vi "ClearSession.vi"(8 "error in (no error)":errorcluster, 11 "Python in":T2) -> (0 "error out":errorcluster, 3 "Arduino":T1)   [LabVIEW 2021]
uses:
  PythonCtrl.ctl
  Processors.ctl
  ArduinoCtrl.ctl
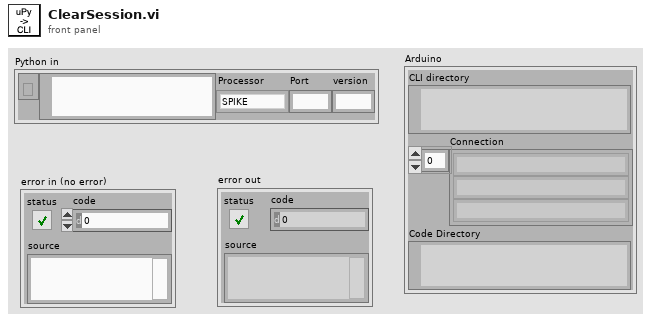
[diagram p1: front panel]
types:
  T1 = typedef "ArduinoCtrl.ctl" = cluster{"CLI directory":path, "Connection":string[], "Code Directory":path}
  T2 = typedef "PythonCtrl.ctl" = cluster{"session":refnum<k35>, "PyPath":path, "Processor":T3, "Port":string, "version":string}
  T3 = typedef "Processors.ctl" = enum16{"SPIKE", "Pi", "Pi_ssh", "OpenMV", "Dunio"}
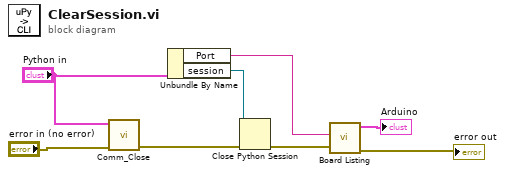
[diagram p0: block diagram]
diagram:
  n1 = call "Comm_Close.vi"("error in (no error)"="error in (no error)", "Python in"="Python in") -> ("error out"=w6:errorcluster)  [unwired: 8 in, 1 out]
  n2 = Unbundle By Name("Python in") -> ("Port"=w4:string, "session"=w7:refnum<k35>)
  n3 = Close Python Session(session in=w7, error in=w6) -> (11:w3:errorcluster)
  n4 = call "Board Listing.vi"("error in"=w3, "desired port"=w4) -> ("error out"=→"error out":errorcluster, "Arduino"=→"Arduino":T1)  [unwired: 7 in, 1 out]
